vi "Main.vi"() -> ()   [LabVIEW 2019]
uses:
  <vilib>/robotics/Kinematics/NI_Kinematics.lvlib
  <vilib>/myRIO/Instrument Drivers/Onboard IO/PWM/typedefs/PWM Configuration.ctl
  <vilib>/myRIO/Instrument Drivers/Onboard IO/PWM/PWM.lvlib
  <vilib>/myRIO/Common/Instrument Driver Framework/myRIO v1.0/PWM/typedefs/PWM Channels Enum.ctl
  <vilib>/myRIO/Common/Instrument Driver Framework/Utilities/typedefs/Generic FPGA Reference.ctl
  <vilib>/myRIO/Common/Instrument Driver Framework/Utilities/typedefs/myRIO v1.0 Reference.ctl
  <vilib>/myRIO/Common/Instrument Driver Framework/Utilities/typedefs/Hardware Version Enum.ctl
  <vilib>/myRIO/Common/Instrument Driver Framework/Utilities/typedefs/myRIO Generic Hardware Reference.ctl
  <vilib>/myRIO/Instrument Drivers/Onboard IO/PWM/typedefs/PWM Reference.ctl
  <vilib>/myRIO/Instrument Drivers/Onboard IO/PWM/vis/Set Duty Cycle and Frequency.vi
  <vilib>/userDefined/High Color/nirio_resource_hc.ctl
  <vilib>/myRIO/Common/Instrument Driver Framework/myRIO v1.0/PWM/vis/myRIO v1.1 Open PWM.vi
  <vilib>/myRIO/Instrument Drivers/Onboard IO/PWM/vis/myRIO PWM Open.xnode
  <vilib>/myRIO/Common/Instrument Driver Framework/Utilities/vis/Is FPGA Ref Available.vi
  <vilib>/myRIO/Express VI/Onboard IO/PWM/PWM Express VI.xnode
  <vilib>/myRIO/Express VI/Onboard Devices/Button/Button Express VI.xnode
  <vilib>/myRIO/Instrument Drivers/Onboard IO/DIO/vis/Read.vi
  <vilib>/myRIO/Instrument Drivers/Onboard IO/DIO/DIO.lvlib
  <vilib>/myRIO/Common/Instrument Driver Framework/myRIO v1.0/DIO/typedefs/DIO Channels Enum.ctl
  <vilib>/myRIO/Common/Instrument Driver Framework/myRIO v1.0/DIO/typedefs/DIO Channels List.ctl
  <vilib>/myRIO/Instrument Drivers/Onboard IO/DIO/typedefs/DIO Reference.ctl
  <vilib>/myRIO/Instrument Drivers/Onboard IO/DIO/vis/myRIO DIO Open.xnode
  <vilib>/myRIO/Common/Instrument Driver Framework/myRIO v1.0/DIO/vis/myRIO v1.1 Open DIO.vi
  <vilib>/robotics/Kinematics/Generate Joint Trajectory (Int).vi
panel:
  out "Time Stamp":timestamp
  in  "Tab Control":enum32{"Trajectory", "Array table"}(tab)
  out "Servo 1":dbl
  out "Servo 1":dbl[](graph)
  out "Servo 2":dbl[](graph)
  out "Servo 3":dbl[](graph)
  out "Servo 4":dbl[](graph)
  out "Servo 5":dbl[](graph)
  out "Servo 6":dbl[](graph)
  out "Servo 2":dbl
  out "Servo 3":dbl
  out "Servo 4":dbl
  out "Servo 5":dbl
  out "Servo 6":dbl
  out "joint position trajectory":dbl[][](array[numeric])
  out "Start position":dbl[](array[numeric])
  out "End position":dbl[](array[numeric])
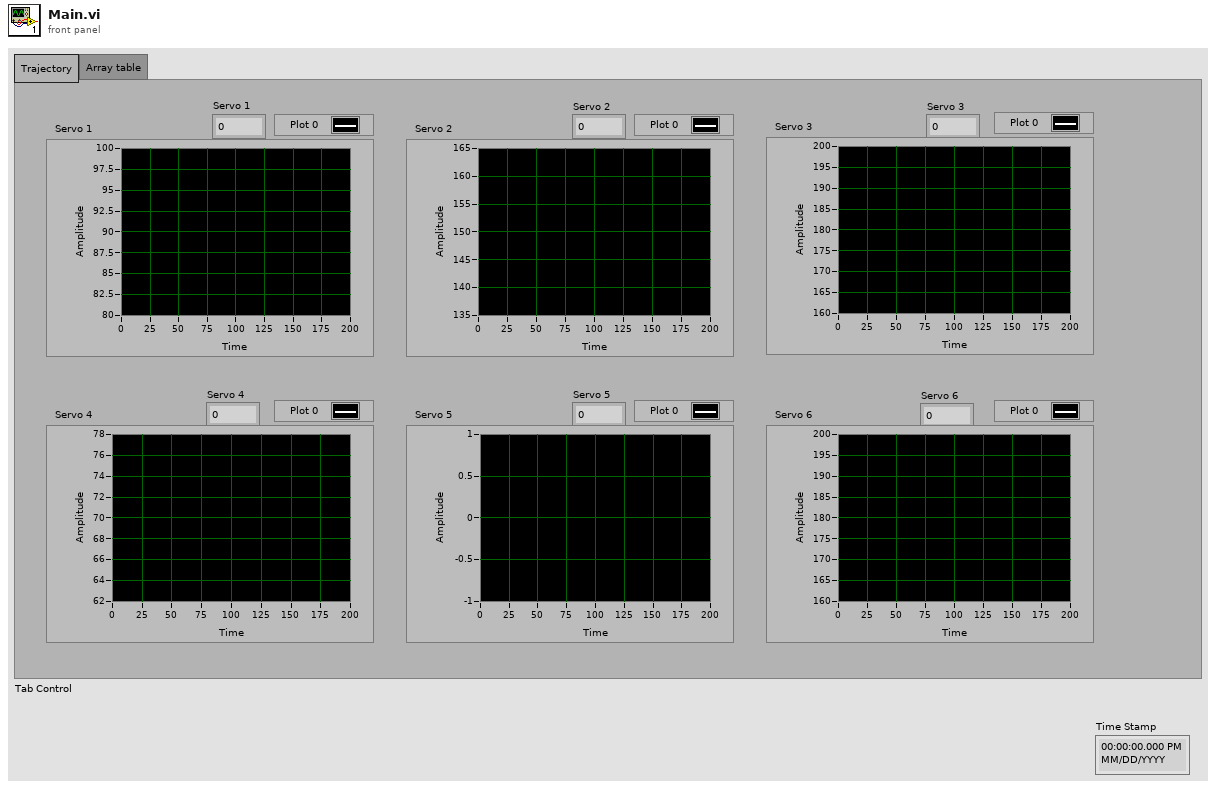
[diagram p1: front panel]
types:
  T1 = typedef "PWM.lvlib/PWM Reference.ctl" = cluster{"myRIO Reference":T2, "PWM Channels Enum":T6, "PWM Configuration":T7}
  T2 = typedef "myRIO Generic Hardware Reference.ctl" = cluster{"myRIO Model":T3, "myRIO Hardware Reference":T4}
  T3 = typedef "Hardware Version Enum.ctl" = enum16{"Unknown", "myRIO-1900", "myRIO-1950", "roboRIO", "NI ELVIS RIO CM", "ELVIS III"}
  T4 = typedef "myRIO v1.0 Reference.ctl" = cluster{"Generic FPGA Reference":T5, "Allow multiple opens":bool}
  T5 = typedef "Generic FPGA Reference.ctl" = refnum<k20>
  T6 = typedef "PWM Channels Enum.ctl" = enum16{"Not Connected", "C/PWM0", "C/PWM1", "A/PWM0", "A/PWM1", "A/PWM2", "A/PWM3", "A/PWM4", "A/PWM5", "A/PWM6", "A/PWM7", "A/PWM8", "A/PWM9", "A/PWM10", "A/PWM11", "A/PWM12", "A/PWM13", "A/PWM14", "A/PWM15", "A/PWM16", "A/PWM17", "A/PWM18", "A/PWM19", "B/PWM0", "B/PWM1", "B/PWM2", "B/PWM3", "B/PWM4", "B/PWM5", "B/PWM6", "B/PWM7", "B/PWM8", "B/PWM9", "B/PWM10", "B/PWM11", "B/PWM12", "B/PWM13", "B/PWM14", "B/PWM15", "B/PWM16", "B/PWM17", "B/PWM18", "B/PWM19", "PWM/PWM0", "PWM/PWM1", "PWM/PWM2", "PWM/PWM3", "PWM/PWM4", "PWM/PWM5", "PWM/PWM6", "PWM/PWM7", "PWM/PWM8", "PWM/PWM9"}
  T7 = typedef "PWM.lvlib/PWM Configuration.ctl" = cluster{"Frequency":dbl, "Duty Cycle":dbl}
  T8 = typedef "nirio_resource_hc.ctl" = tag
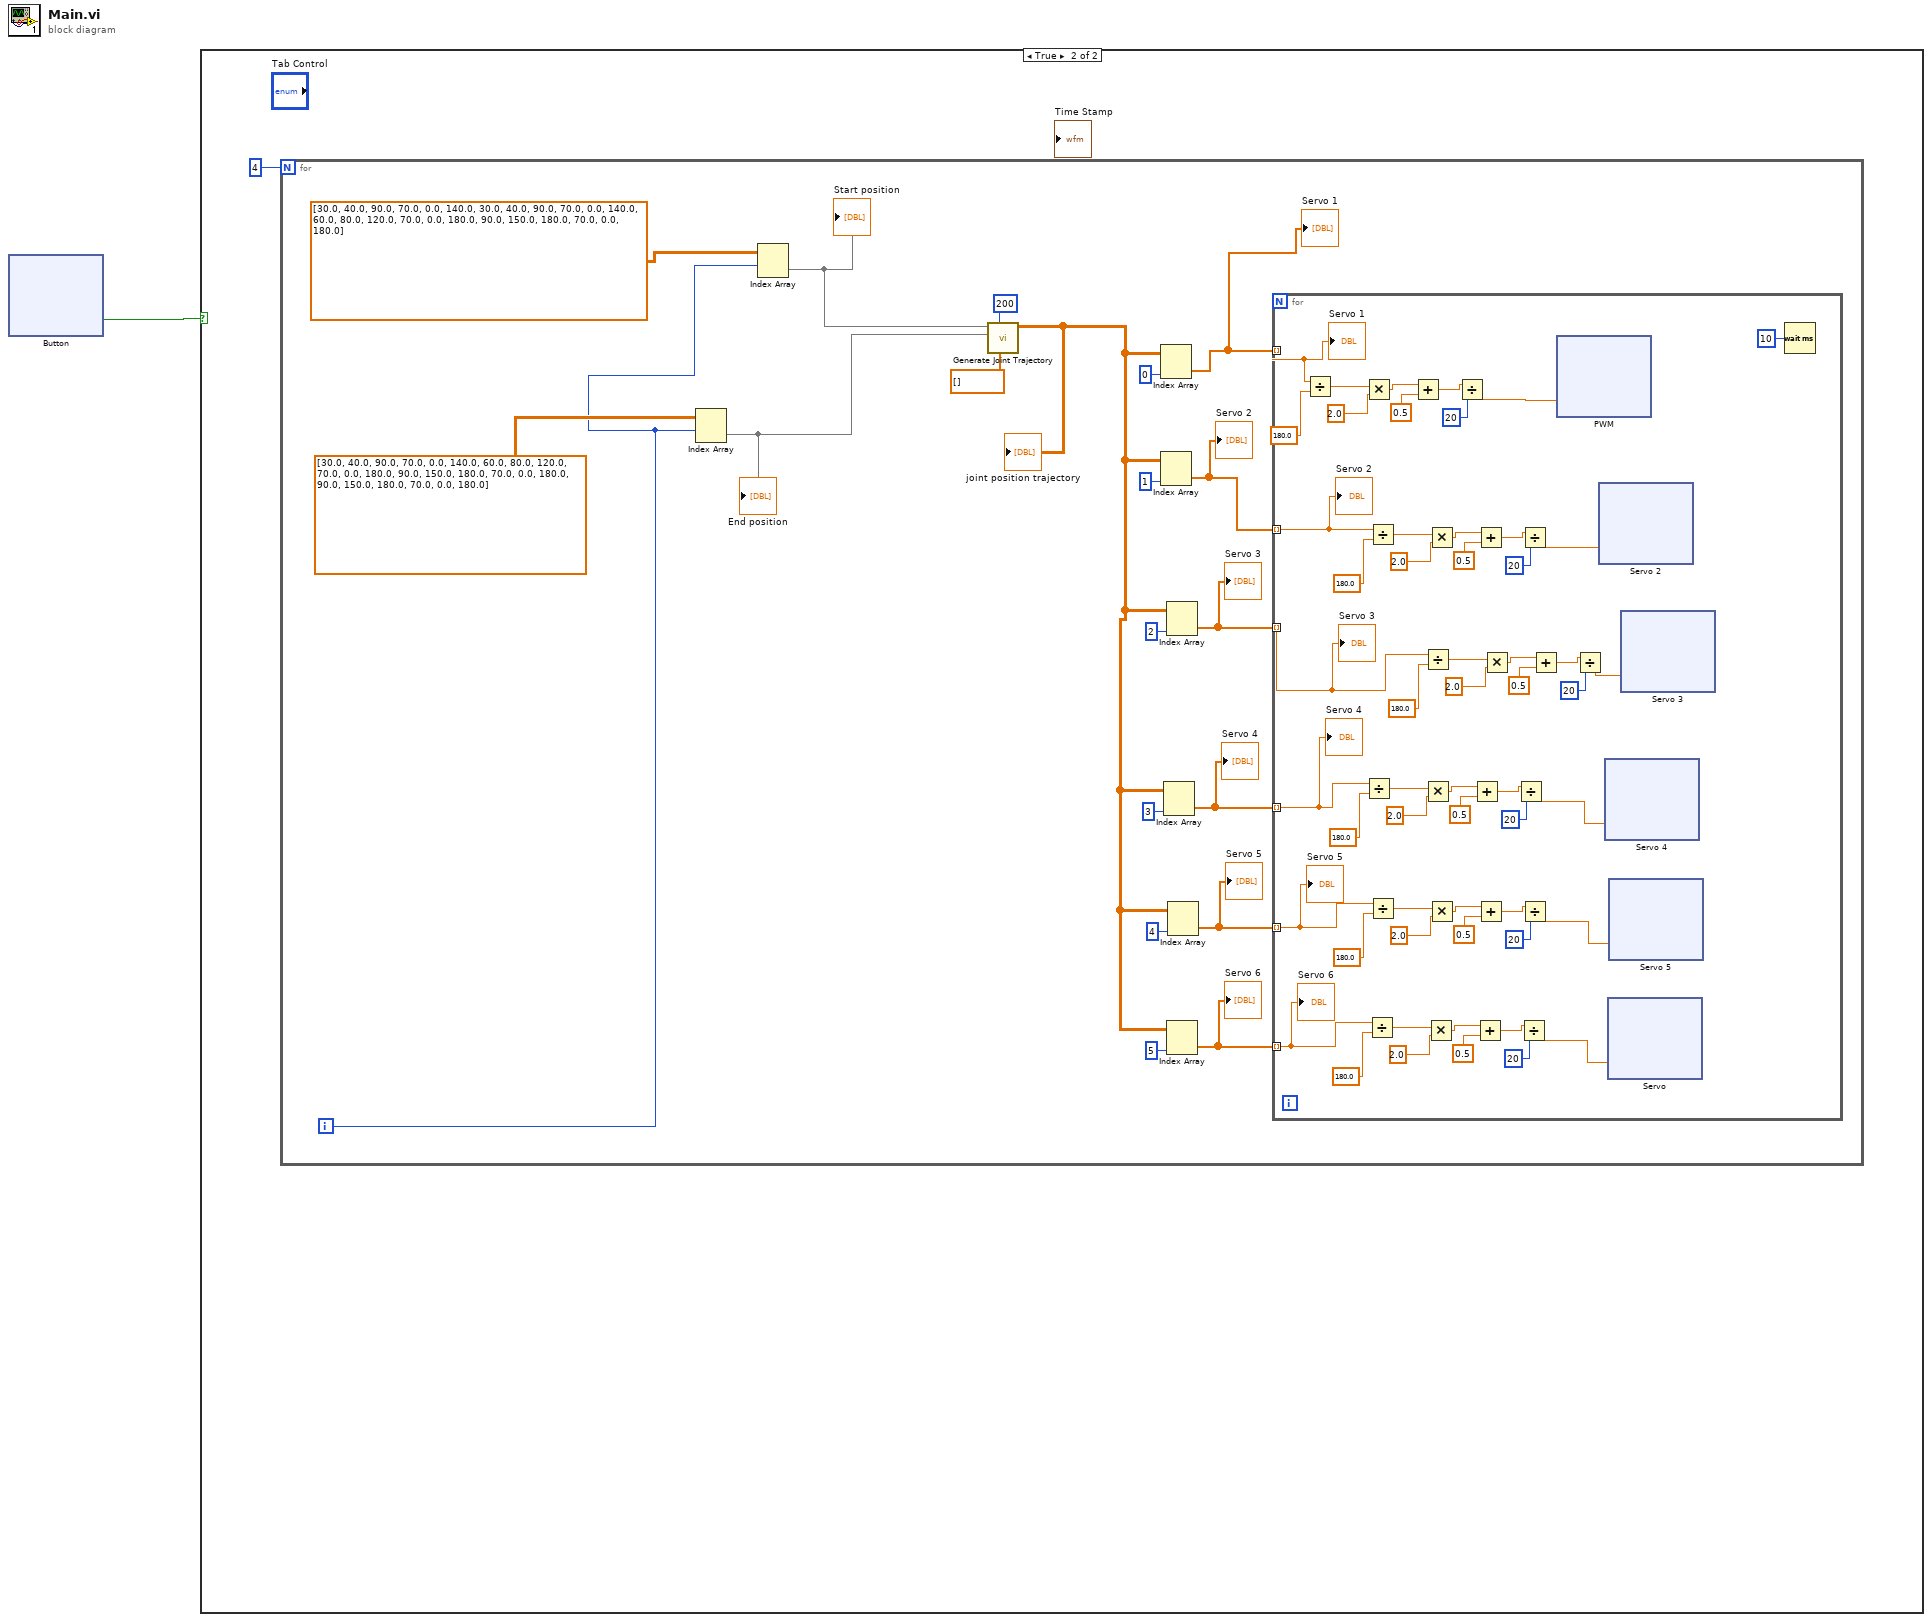
[diagram p0: block diagram]
diagram:
  n1 = xnode "Button"() -> ("Value"=w1:bool)  [unwired: 1 in, 1 out]
  n2 = case shown="True" w1 {
    frame False {
    }
    frame True {
      n3 = for {
        N: 4 -> [_]
        i -> [w15]
        n4 = Index Array(array=dbl[][] [[30.0, 40.0, 90.0, 70.0, 0.0, 140.0], [60.0, 80.0, 120.0, 70.0, 0.0, 180.0], [90.0, 150.0, 180.0, 70.0, 0.0, 180.0], [90.0, 150.0, 180.0, 70.0, 0.0, 180.0]] ("start joint velocities"), index (row)=w15) -> (element=w16:dbl[])  [unwired: 1 in]
        "End position" <- w16
        n5 = Index Array(array=dbl[][] [[30.0, 40.0, 90.0, 70.0, 0.0, 140.0], [30.0, 40.0, 90.0, 70.0, 0.0, 140.0], [60.0, 80.0, 120.0, 70.0, 0.0, 180.0], [90.0, 150.0, 180.0, 70.0, 0.0, 180.0]] ("start joint positions"), index (row)=w15) -> (element=w17:dbl[])  [unwired: 1 in]
        "Start position" <- w17
        n6 = call-poly <vilib>:"Generate Joint Trajectory.vi"("start joint velocities"=dbl[] [], "intermediate points"=200, "end joint positions"=w16, "start joint positions"=w17) -> ("joint position trajectory"=w3:dbl[][])  [unwired: 4 in, 3 out]
        "joint position trajectory" <- w3
        n7 = Index Array(array=w3, index (col)=0 ("disabled index (col)")) -> (element=w20:dbl[])  [unwired: 1 in]
        "Servo 1" <- w20
        n8 = Index Array(array=w3, index (col)=1 ("disabled index (col)")) -> (element=w10:dbl[])  [unwired: 1 in]
        "Servo 2" <- w10
        n9 = Index Array(array=w3, index (col)=3) -> (element=w8:dbl[])  [unwired: 1 in]
        "Servo 4" <- w8
        n10 = Index Array(array=w3, index (col)=2) -> (element=w11:dbl[])  [unwired: 1 in]
        "Servo 3" <- w11
        n11 = Index Array(array=w3, index (col)=5) -> (element=w4:dbl[])  [unwired: 1 in]
        "Servo 6" <- w4
        n12 = Index Array(array=w3, index (col)=4) -> (element=w7:dbl[])  [unwired: 1 in]
        "Servo 5" <- w7
        n13 = for {
          tunnel: w20 -> [w28] mode=indexing
          tunnel: w10 -> [w27] mode=indexing
          tunnel: w11 -> [w26] mode=indexing
          tunnel: w8 -> [w25] mode=indexing
          tunnel: w7 -> [w24] mode=indexing
          tunnel: w4 -> [w23] mode=indexing
          n14 = Divide(x=w28, y=180.0) -> (x/y=w72:dbl)
          n15 = Multiply(x=w72, y=2.0) -> (x*y=w76:dbl)
          n16 = Divide(x=w25, y=180.0) -> (x/y=w47:dbl)
          n17 = Divide(x=w23, y=180.0) -> (x/y=w31:dbl)
          n18 = Divide(x=w27, y=180.0) -> (x/y=w64:dbl)
          n19 = Divide(x=w24, y=180.0) -> (x/y=w42:dbl)
          n20 = Add(x=w76, y=0.5) -> (x+y=w74:dbl)
          n21 = Divide(x=w26, y=180.0) -> (x/y=w58:dbl)
          n22 = Multiply(x=w47, y=2.0) -> (x*y=w51:dbl)
          n23 = Multiply(x=w31, y=2.0) -> (x*y=w35:dbl)
          n24 = Multiply(x=w64, y=2.0) -> (x*y=w68:dbl)
          n25 = Multiply(x=w42, y=2.0) -> (x*y=w38:dbl)
          n26 = Divide(x=w74, y=20) -> (x/y=w71:dbl)
          n27 = Add(x=w51, y=0.5) -> (x+y=w49:dbl)
          n28 = Add(x=w35, y=0.5) -> (x+y=w33:dbl)
          n29 = Add(x=w68, y=0.5) -> (x+y=w66:dbl)
          n30 = Add(x=w38, y=0.5) -> (x+y=w40:dbl)
          n31 = Multiply(x=w58, y=2.0) -> (x*y=w54:dbl)
          n32 = Divide(x=w49, y=20) -> (x/y=w46:dbl)
          n33 = Divide(x=w33, y=20) -> (x/y=w30:dbl)
          n34 = Divide(x=w66, y=20) -> (x/y=w63:dbl)
          n35 = Divide(x=w40, y=20) -> (x/y=w43:dbl)
          n36 = Add(x=w54, y=0.5) -> (x+y=w56:dbl)
          n37 = xnode "PWM"("Duty Cycle"=w71) -> ()  [unwired: 1 in, 1 out]
          n38 = Divide(x=w56, y=20) -> (x/y=w59:dbl)
          n39 = xnode "Servo 2"("Duty Cycle"=w63) -> ()  [unwired: 1 in, 1 out]
          n40 = xnode "Servo 4"("Duty Cycle"=w46) -> ()  [unwired: 1 in, 1 out]
          n41 = xnode "Servo"("Duty Cycle"=w30) -> ()  [unwired: 1 in, 1 out]
          n42 = xnode "Servo 5"("Duty Cycle"=w43) -> ()  [unwired: 1 in, 1 out]
          n43 = xnode "Servo 3"("Duty Cycle"=w59) -> ()  [unwired: 1 in, 1 out]
          n44 = Wait (ms)(milliseconds to wait=u32 10) -> ()  [unwired: 1 out]
          "Servo 1" <- w28
          "Servo 2" <- w27
          "Servo 3" <- w26
          "Servo 4" <- w25
          "Servo 5" <- w24
          "Servo 6" <- w23
        }
      }
    }
  }
